vi "闹钟（任意）.vi"(5 "设置时间":timestamp, 7 "启用":bool=TRUE) -> (6 "时间到脉冲":bool, 8 "当前时间":timestamp)   [LabVIEW 2012]
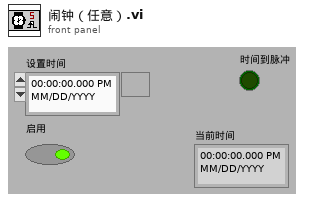
[diagram p1: front panel]
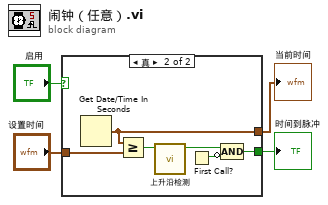
[diagram p0: block diagram]
diagram:
  n1 = case shown="真" "启用" {
    tunnel: "设置时间" -> [_ w7]
    tunnel: [_ w10] -> w2
    tunnel: [_ w5] -> w1
    frame False {
    }
    frame True {
      n2 = Get Date/Time In Seconds() -> (seconds since 1Jan1904=w5:timestamp)
      n3 = Greater Or Equal?(x=w5, y=w7) -> (x >= y?=w8:bool)
      n4 = call "上升沿检测.vi"("input"=w8) -> ("output"=w6:bool)  [unwired: 9 in, 1 out]
      n5 = First Call?() -> (First Call?: T/F=w9:bool)
      n6 = Compound Arithmetic op=AND(w6, invert w9) -> (w10:bool)
    }
  }
  "时间到脉冲" <- w2
  "当前时间" <- w1
